vi "GetCellFormulae.vi"(11 "XML":string) -> (2 "Type":string[](array[string]), 3 "Value":string[](array[string]))   [LabVIEW 2013]
uses:
  XML.lvlib
  <vilib>/xml/NI_XML.lvlib
  <resource>/objmgr/DOMUserDefRef.rc
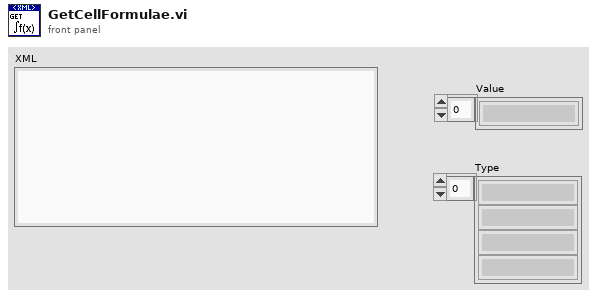
[diagram p1: front panel]
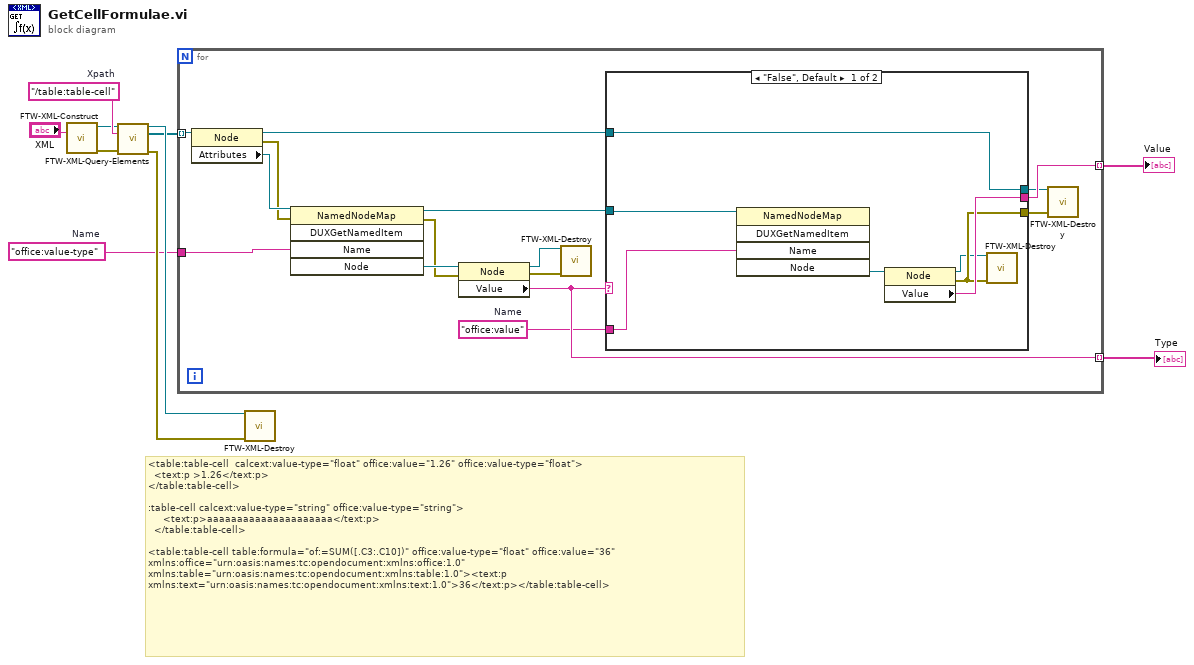
[diagram p0: block diagram]
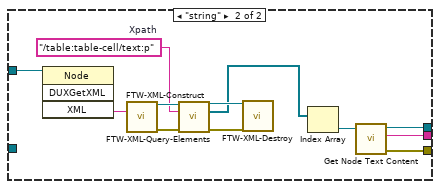
[diagram p2: hidden frame]
diagram:
  w2 = "office:value-type"  # Name
  w7 = "/table:table-cell"  # Xpath
  # "<table:table-cell  calcext:value-type=\"float\" office:value=\"1.26\" office:value-type=\"float\">\n  <text:p >1.26</text:p>\n</table:table-cell>\n\n:table-cell calcext:value-type=\"string\" office:value-type=\"string\">           \n     <text:p>aaaaaaaaaaaaaaaaaaaaa</text:p>\n  </table:table-cell>\n\n<table:table-cell table:formula=\"of:=SUM([.C3:.C10])\" office:value-type=\"float\" office:value=\"36\" xmlns:office=\"urn:oasis:names:tc:opendocument:xmlns:office:1.0\" xmlns:table=\"urn:oasis:names:tc:opendocument:xmlns:table:1.0\"><text:p xmlns:text=\"urn:oasis:names:tc:opendocument:xmlns:text:1.0\">36</text:p></table:table-cell>"
  n1 = call "FTW-XML-Construct.vi"("XML String"="XML") -> ("XML Document"=w5:refnum<k20>, "error out"=w6:errorcluster)  [unwired: 13 in]
  n2 = call "FTW-XML-Query-Elements.vi"("XML Node"=w5, "XPath Query"=w7, "error in"=w6) -> ("XML Node out"=w10:refnum<k20>, "Matching Nodes"=w8:refnum<k20>[], "error out"=w9:errorcluster)  [unwired: 9 in, 1 out]
  n3 = for {
    tunnel: [w25] -> w3 mode=indexing
    tunnel: w8 -> [w22] mode=indexing
    tunnel: w2 -> [w18]
    tunnel: [w13] -> w1 mode=indexing
    w11 = "office:value"  # Name
    n4 = property class="Node"(reference=w22) -> (reference out=w20:refnum<k20>, error out=w19:errorcluster, "Attributes"=w21:refnum<k20>)  [unwired: 1 in]
    n5 = invoke class="NamedNodeMap" method="DUXGetNamedItem"(reference=w21, error in=w19, "Name"=w18) -> (reference out=w12:refnum<k20>, error out=w14:errorcluster, "Node"=w17:refnum<k20>)  [unwired: 2 in, 2 out]
    n6 = property class="Node"(reference=w17, error in=w14) -> (reference out=w15:refnum<k20>, error out=w16:errorcluster, "Value"=w13:string)
    n7 = call "FTW-XML-Destroy.vi"("XML Node"=w15, "error in"=w16) -> ()  [unwired: 13 in, 1 out]
    n8 = case shown="\"False\", Default" w13 {
      tunnel: [w28 w44] -> w25
      tunnel: [w27 w43] -> w24
      tunnel: [w31 w42] -> w23
      tunnel: w20 -> [w31 w41]
      tunnel: w12 -> [w32 _]
      tunnel: w11 -> [w30 _]
      frame "False", Default {
        n9 = invoke class="NamedNodeMap" method="DUXGetNamedItem"(reference=w32, "Name"=w30) -> ("Node"=w29:refnum<k20>)  [unwired: 3 in, 4 out]
        n10 = property class="Node"(reference=w29) -> (reference out=w26:refnum<k20>, error out=w27:errorcluster, "Value"=w28:string)  [unwired: 1 in]
        n11 = call "FTW-XML-Destroy.vi"("XML Node"=w26, "error in"=w27) -> ()  [unwired: 13 in, 1 out]
      }
      frame "string" {
        w33 = "/table:table-cell/text:p"  # Xpath
        n12 = invoke class="Node" method="DUXGetXML"(reference=w41) -> ("XML"=w40:string)  [unwired: 3 in, 3 out]
        n13 = call "FTW-XML-Construct.vi"("XML String"=w40) -> ("XML Document"=w39:refnum<k20>, "error out"=w38:errorcluster)  [unwired: 13 in]
        n14 = call "FTW-XML-Query-Elements.vi"("XML Node"=w39, "XPath Query"=w33, "error in"=w38) -> ("XML Node out"=w36:refnum<k20>, "Matching Nodes"=w35:refnum<k20>[], "error out"=w37:errorcluster)  [unwired: 9 in, 1 out]
        n15 = call "FTW-XML-Destroy.vi"("XML Node"=w36, "error in"=w37) -> ()  [unwired: 13 in, 1 out]
        n16 = Index Array(array=w35) -> (element=w34:refnum<k20>)  [unwired: 1 in]
        n17 = call <vilib>:"Get Node Text Content.vi"("node in"=w34) -> ("error out"=w43:errorcluster, "node text"=w44:string, "node out"=w42:refnum<k20>)  [unwired: 8 in]
      }
    }
    n18 = call "FTW-XML-Destroy.vi"("XML Node"=w23, "error in"=w24) -> ()  [unwired: 13 in, 1 out]
  }
  "Value" <- w3
  "Type" <- w1
  n19 = call "FTW-XML-Destroy.vi"("XML Node"=w10, "error in"=w9) -> ()  [unwired: 13 in, 1 out]
